vi "IntakeTeleop.vi"(11 "Left Y Axis":dbl) -> ()   [LabVIEW 2017]
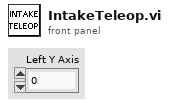
[diagram p1: front panel]
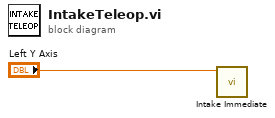
[diagram p0: block diagram]
diagram:
  n1 = call "Intake Immediate.vi"("Speed"="Left Y Axis") -> ()  [unwired: 10 in, 1 out]
